vi "TagsToArray.vi"(1 "Tags":string) -> (0 "Array":string[](array[string]))   [LabVIEW 2012]
doc: "Converts all found XML tags to an array. Returns both opening and closing tags"
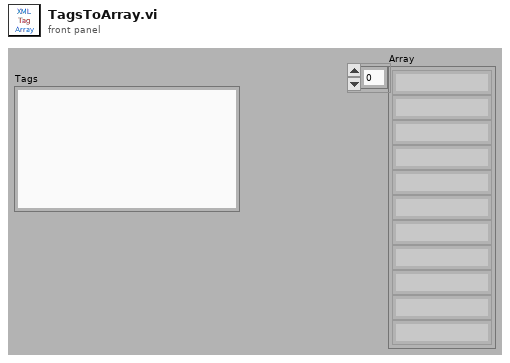
[diagram p1: front panel]
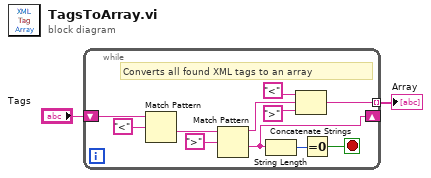
[diagram p0: block diagram]
diagram:
  n1 = while {
    shift-right: [w7] -> _
    shift-left: "Tags" -> [w13]
    tunnel: [w8] -> w1 mode=indexing
    stop <- w5 stop-if-true
    # "Converts all found XML tags to an array"
    n2 = Match Pattern(string=w13, regular expression="<") -> (after substring=w11:string)  [unwired: 1 in, 3 out]
    n3 = Match Pattern(string=w11, regular expression=">") -> (before substring=w4:string, after substring=w7:string)  [unwired: 1 in, 2 out]
    n4 = String Length(string=w7) -> (length=w6:i32)
    n5 = Concatenate Strings("<" ("string"), w4, ">" ("string")) -> (w8:string)
    n6 = Equal To 0?(x=w6) -> (x = 0?=w5:bool)
  }
  "Array" <- w1
